vi "Pcre2GetMatchOffsOfSubstrNumFromOvector8.vi"(8 "error in":errorcluster, 9 "Number":i32, 10 "MatchResult":i32=-1, 11 "pOvector":u64) -> (0 "error out":errorcluster, 1 "OffsetPastMatch":i32, 2 "MatchOffset":i32, 3 "pOvektor":u64 format="%.0x")   [LabVIEW 2021, in "libpcre2-8.lvlib"]
uses:
  libpcre2-8.lvlib
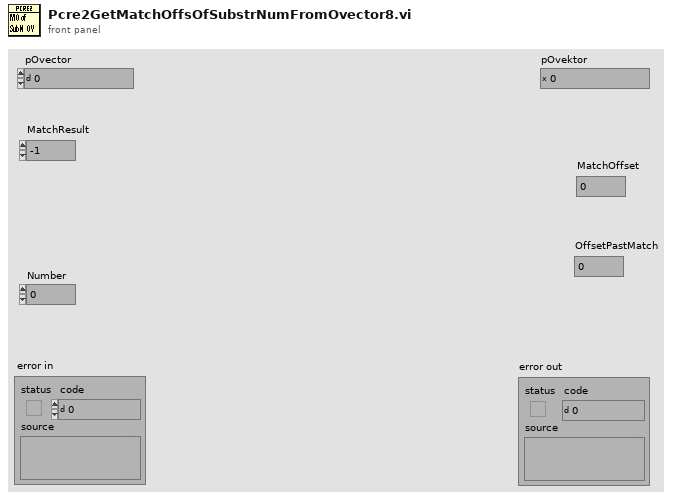
[diagram p1: front panel]
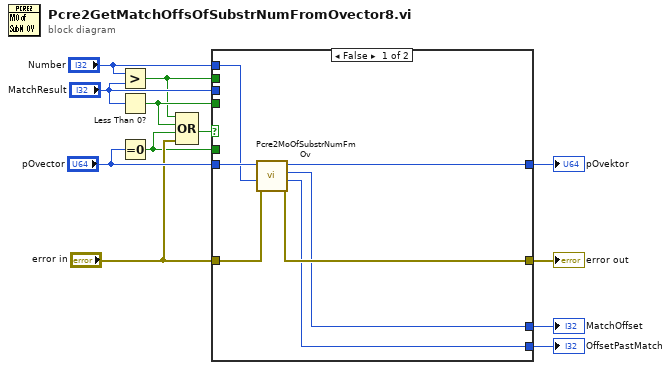
[diagram p0: block diagram]
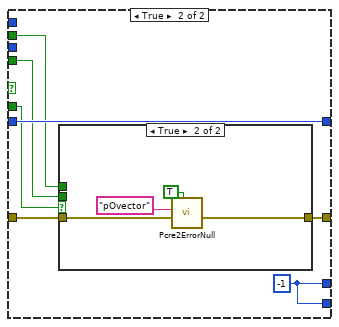
[diagram p2: hidden frame]
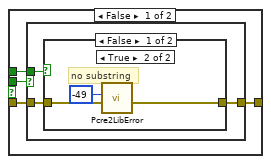
[diagram p3: hidden frame]
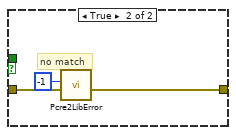
[diagram p5: hidden frame]
diagram:
  n1 = Greater?(x="Number", y="MatchResult") -> (0:w1:bool)
  n2 = Less Than 0?(x="MatchResult") -> (x < 0?=w5:bool)
  n3 = Equal To 0?(x="pOvector") -> (x = 0?=w4:bool)
  n4 = Compound Arithmetic op=OR(w1, w5, w4, "error in") -> (w7:bool)
  n5 = case shown="False" w7 {
    tunnel: "error in" -> [w16 w23]
    tunnel: [w15 w25] -> w12
    tunnel: "pOvector" -> [w18 w26]
    tunnel: [w19 w26] -> w11
    tunnel: [w13 w20] -> w9
    tunnel: [w14 w20] -> w8
    tunnel: "MatchResult" -> [_ _]
    tunnel: w5 -> [_ w22]
    tunnel: w4 -> [_ w24]
    tunnel: "Number" -> [w17 _]
    tunnel: w1 -> [_ w21]
    frame False {
      n6 = call "Pcre2MoOfSubstrNumFmOv.vi"("error in"=w16, "Number"=w17, "pOvector"=w18) -> ("error out"=w15:errorcluster, "OffsetPastMatch"=w14:i32, "MatchOffset"=w13:i32, "pOvektor"=w19:u64)  [unwired: 5 in]
    }
    frame True {
      w20 = -1
      n7 = case shown="True" w24 {
        tunnel: w23 -> [w29 w44]
        tunnel: [w28 w43] -> w25
        tunnel: w22 -> [w30 _]
        tunnel: w21 -> [w27 _]
        frame False {
          n8 = case shown="False" w30 {
            tunnel: w29 -> [w32 w40]
            tunnel: [w31 w39] -> w28
            tunnel: w27 -> [w33 _]
            frame False {
              n9 = case shown="True" w33 {
                tunnel: w32 -> [w34 w36]
                tunnel: [w34 w37] -> w31
                frame False {
                }
                frame True {
                  # "no substring"
                  n10 = call "Pcre2LibError.vi"("error in"=w36, "ErrorCode"=-49) -> ("error out"=w37:errorcluster)  [unwired: 9 in]
                }
              }
            }
            frame True {
              # "no match"
              n11 = call "Pcre2LibError.vi"("error in"=w40, "ErrorCode"=-1) -> ("error out"=w39:errorcluster)  [unwired: 9 in]
            }
          }
        }
        frame True {
          n12 = call "Pcre2ErrorNull.vi"("IsPointer? (F)"=TRUE, "error in"=w44, "What"="pOvector") -> ("error out"=w43:errorcluster)  [unwired: 8 in]
        }
      }
    }
  }
  "pOvektor" <- w11
  "error out" <- w12
  "MatchOffset" <- w9
  "OffsetPastMatch" <- w8
